vi "Translate.vi"(0 "Speed":i16, 11 "Turn":i16) -> (4 "Right Motor Speed":i16, 15 "Left Motor Speed":i16)   [LabVIEW 2009]
doc: "This VI takes in Speed and Turn values and converts them into wheel speeds.\nNOTE : Turn value of 0 indicates that the robot will go straight"
panel:
  in  "Min axix turn speed":i16=6
  in  "Max axix turn speed":i16=30
  in  "Wheel Diameter 2":dbl=0.4191 caption="Wheel Diameter=r(m)"
  out "Global wl":dbl
  out "Global wr":dbl
  out "wl":dbl caption="Left wheel angular velocity=wl(R/s)"
  out "wr":dbl caption="Right wheel angular velocity=wr(R/s)"
  in  "Wheel Diameter":dbl=0.21 caption="Wheel Radius=r(m)"
  in  "Distance Between wheels":dbl=0.6096 caption="Distance between wheels=L(m)"
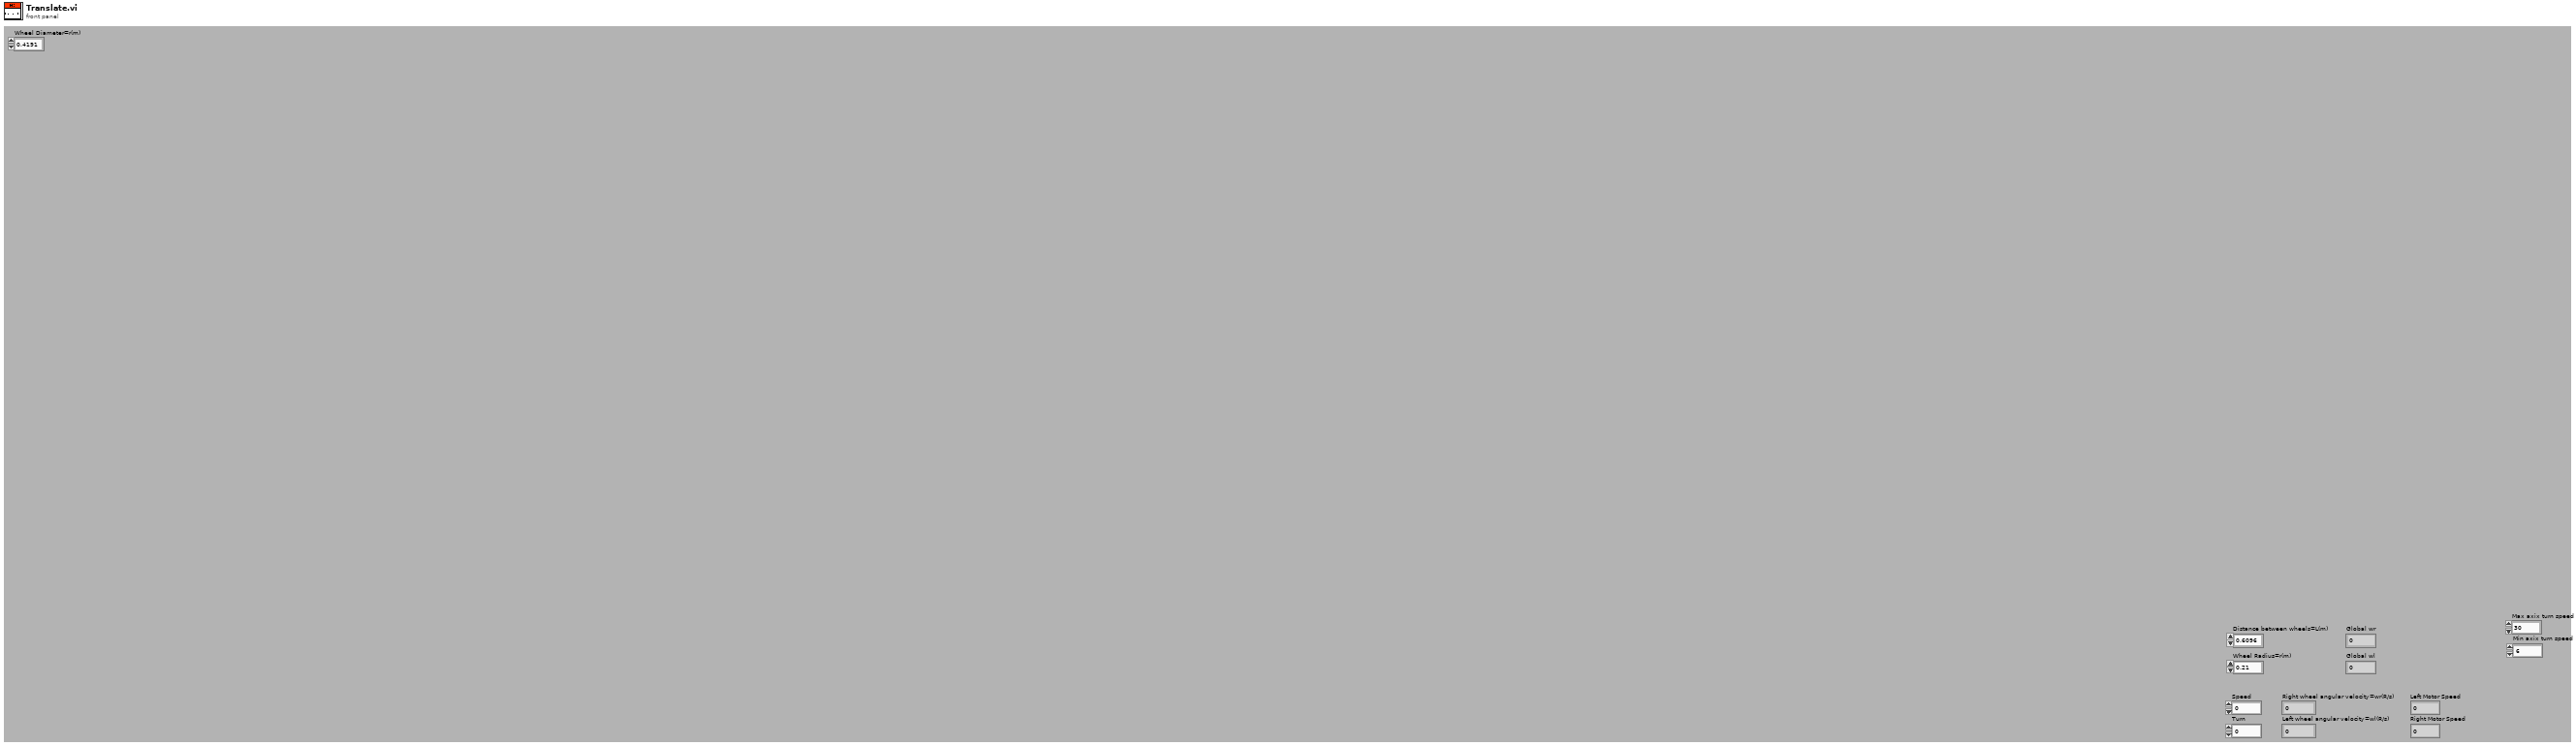
[diagram p1: front panel]
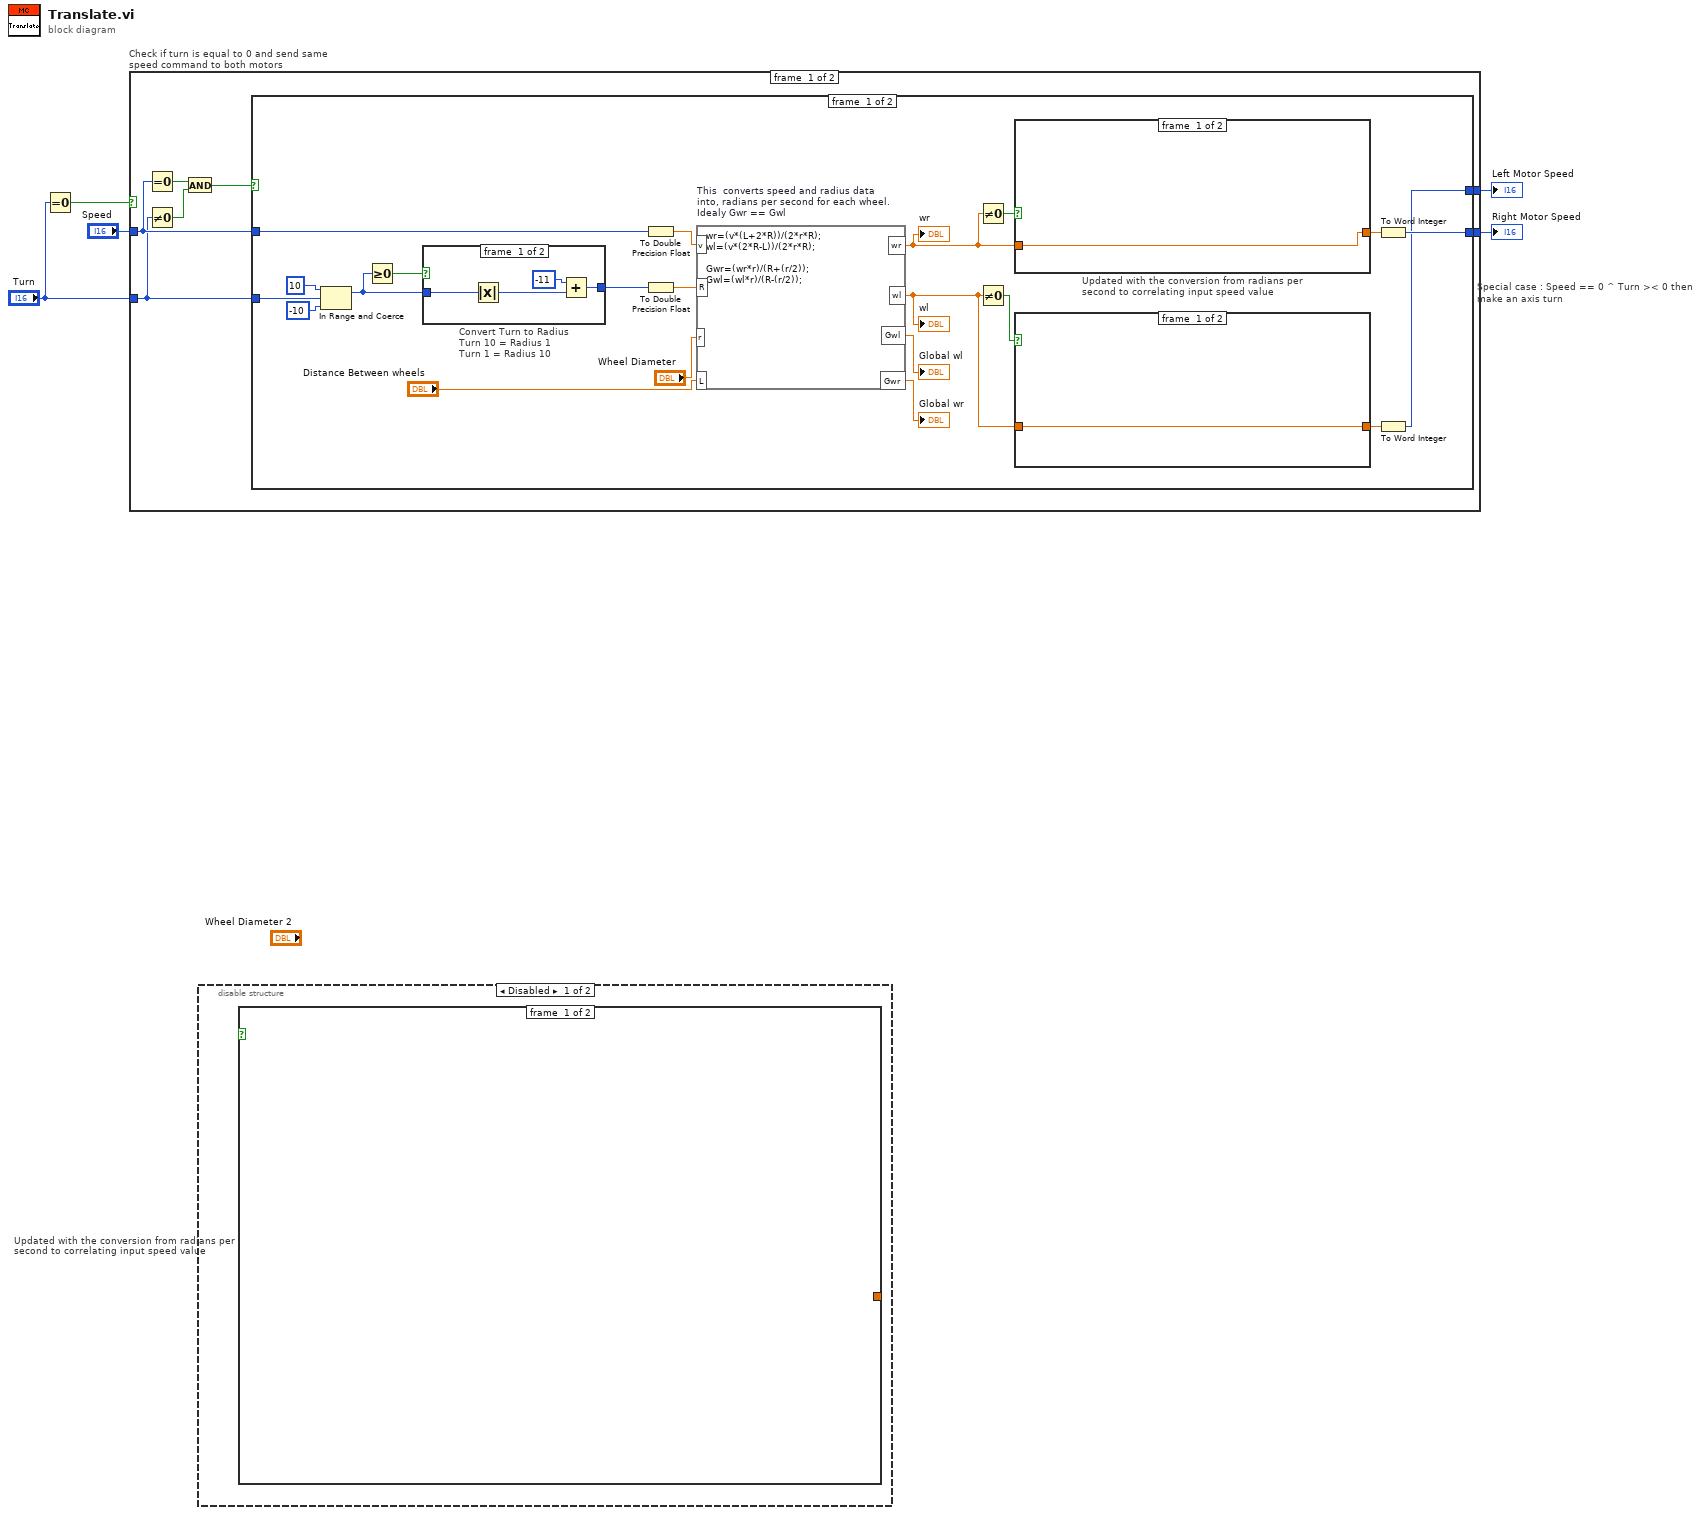
[diagram p0: block diagram]
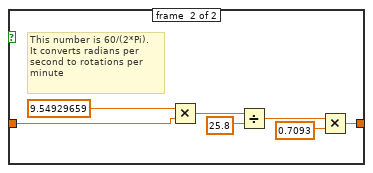
[diagram p2: hidden frame]
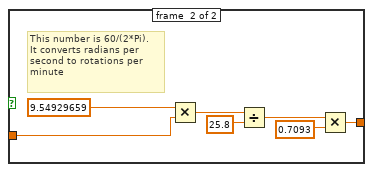
[diagram p3: hidden frame]
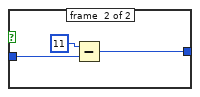
[diagram p4: hidden frame]
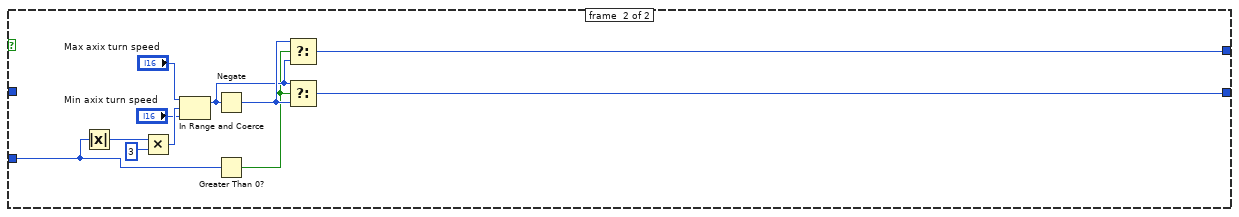
[diagram p5: hidden frame]
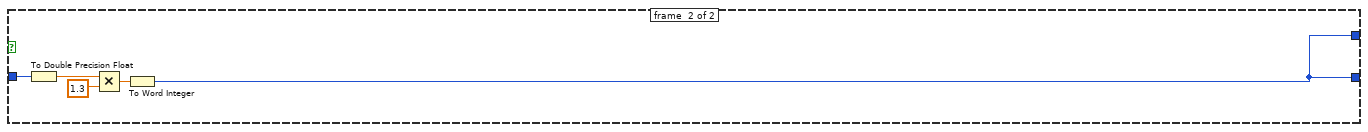
[diagram p6: hidden frame]
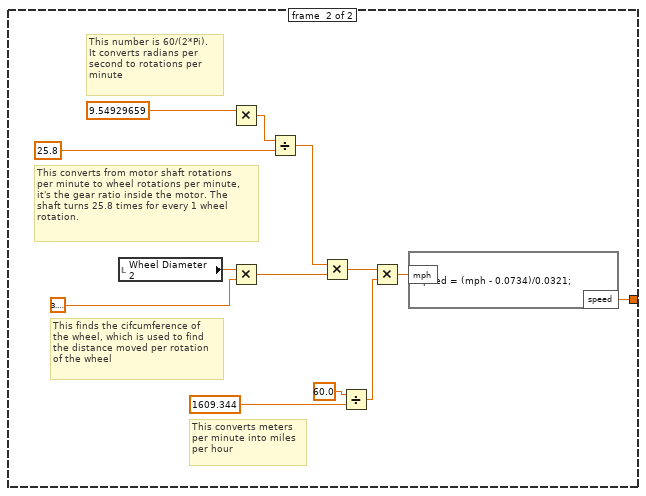
[diagram p7: hidden frame]
diagram:
  n1 = Equal To 0?(x="Turn") -> (x = 0?=w4:bool)
  n2 = case "Check if turn is equal to 0 and send same speed command to both motors" shown="False" w4 {
    tunnel: "Turn" -> [w8 _]
    tunnel: "Speed" -> [w10 w72]
    tunnel: [w12 w69] -> w2
    tunnel: [w11 w69] -> w1
    frame #0 {
      n3 = Equal To 0?(x=w10) -> (x = 0?=w9:bool)
      n4 = Not Equal To 0?(x=w8) -> (x != 0?=w6:bool)
      n5 = And(x=w9, y=w6) -> (x .and. y?=w7:bool)
      n6 = case "Special case : Speed == 0 ^ Turn >< 0 then make an axis turn" shown="False" w7 {
        tunnel: w8 -> [w27 w65]
        tunnel: w10 -> [w17 _]
        tunnel: [w15 w67] -> w12
        tunnel: [w13 w66] -> w11
        frame #0 {
          n7 = In Range and Coerce(upper limit=i16 10, x=w27, lower limit=i16 -10) -> (coerced(x)=w24:i16)  [unwired: 1 out]
          n8 = Greater Or Equal To 0?(x=w24) -> (x >= 0?=w28:bool)
          n9 = case "Convert Turn to Radius\nTurn 10 = Radius 1\nTurn 1 = Radius 10" shown="False" w28 {
            tunnel: w24 -> [w51 w56]
            tunnel: [w50 w54] -> w23
            frame #0 {
              n10 = Absolute Value(x=w51) -> (abs(x)=w52:i16)
              n11 = Add(x=i16 -11, y=w52) -> (x+y=w50:i16)
            }
            frame #1 {
              n12 = Subtract(x=i16 11, y=w56) -> (x-y=w54:i16)
            }
          }
          n13 = To Double Precision Float(number=w17) -> (double precision float=w18:dbl)
          n14 = To Double Precision Float(number=w23) -> (double precision float=w29:dbl)
          n15 = formula code="wr=(v*(L+2*R))/(2*r*R);\nwl=(v*(2*R-L))/(2*r*R);\n\nGwr=(wr*r)/(R+(r/2));\nGwl=(wl*r)/(R-(r/2));" "This  converts speed and radius data \ninto, radians per second for each wheel.\nIdealy Gwr == Gwl"("v"=w18, "R"=w29, "r"="Wheel Diameter", "L"="Distance Between wheels") -> ("wr"=w21:dbl, "wl"=w19:dbl, "Gwr"=→"Global wr":dbl, "Gwl"=→"Global wl":dbl)
          "wr" <- w21
          "wl" <- w19
          n16 = Not Equal To 0?(x=w21) -> (x != 0?=w22:bool)
          n17 = Not Equal To 0?(x=w19) -> (x != 0?=w20:bool)
          n18 = case "Updated with the conversion from radians per second to correlating input speed value" shown="True" w22 {
            tunnel: w21 -> [w42 w44]
            tunnel: [w42 w43] -> w16
            frame #0 {
            }
            frame #1 {
              # "This number is 60/(2*Pi). \nIt converts radians per \nsecond to rotations per \nminute"
              n19 = Multiply(x=9.54929659, y=w44) -> (x*y=w47:dbl)
              n20 = Divide(x=w47, y=25.8) -> (x/y=w45:dbl)
              n21 = Multiply(x=w45, y=0.7093 ("x")) -> (x*y=w43:dbl)
            }
          }
          n22 = case shown="True" w20 {
            tunnel: w19 -> [w34 w36]
            tunnel: [w34 w35] -> w14
            frame #0 {
            }
            frame #1 {
              # "This number is 60/(2*Pi). \nIt converts radians per \nsecond to rotations per \nminute"
              n23 = Multiply(x=9.54929659, y=w36) -> (x*y=w39:dbl)
              n24 = Divide(x=w39, y=25.8) -> (x/y=w37:dbl)
              n25 = Multiply(x=w37, y=0.7093 ("x")) -> (x*y=w35:dbl)
            }
          }
          n26 = To Word Integer(number=w16) -> (16bit integer=w15:i16)
          n27 = To Word Integer(number=w14) -> (16bit integer=w13:i16)
        }
        frame #1 {
          n28 = Absolute Value(x=w65) -> (abs(x)=w63:i16)
          n29 = Multiply(x=w63, y=i16 3) -> (x*y=w61:i16)
          n30 = In Range and Coerce(upper limit="Max axix turn speed", x=w61, lower limit="Min axix turn speed") -> (coerced(x)=w60:i16)  [unwired: 1 out]
          n31 = Negate(x=w60) -> (-x=w62:i16)
          n32 = Greater Than 0?(x=w65) -> (x > 0?=w57:bool)
          n33 = Select(t=w62, s=w57, f=w60) -> (s? t:f=w66:i16)
          n34 = Select(t=w60, s=w57, f=w62) -> (s? t:f=w67:i16)
        }
      }
    }
    frame #1 {
      n35 = To Double Precision Float(number=w72) -> (double precision float=w68:dbl)
      n36 = Multiply(x=w68, y=1.3) -> (x*y=w70:dbl)
      n37 = To Word Integer(number=w70) -> (16bit integer=w69:i16)
    }
  }
  "Right Motor Speed" <- w2
  "Left Motor Speed" <- w1
  n38 = disable-structure shown="Disabled" {
    frame #0 {
      n39 = case "Updated with the conversion from radians per second to correlating input speed value" shown="True" {
        selector: _ -> [_ _]
        tunnel: [_ w73] -> _
        frame #0 {
        }
        frame #1 {
          # "This converts meters\nper minute into miles\nper hour"
          # "This finds the cifcumference of\nthe wheel, which is used to find \nthe distance moved per rotation\nof the wheel"
          # "This converts from motor shaft rotations \nper minute to wheel rotations per minute,\nit's the gear ratio inside the motor. The \nshaft turns 25.8 times for every 1 wheel \nrotation."
          # "This number is 60/(2*Pi). \nIt converts radians per \nsecond to rotations per \nminute"
          n40 = local read "Wheel Diameter 2"() -> (w80:dbl)
          n41 = Multiply(x=9.54929659) -> (x*y=w84:dbl)  [unwired: 1 in]
          n42 = Multiply(x=w80, y=3.141592653589793) -> (x*y=w79:dbl)
          n43 = Divide(x=w84, y=25.8) -> (x/y=w82:dbl)
          n44 = Multiply(x=w82, y=w79) -> (x*y=w78:dbl)
          n45 = Divide(x=60.0, y=1609.344) -> (x/y=w75:dbl)
          n46 = Multiply(x=w78, y=w75) -> (x*y=w74:dbl)
          n47 = formula code="speed = (mph - 0.0734)/0.0321;"("mph"=w74) -> ("speed"=w73:dbl)
        }
      }
    }
    frame #1 {
    }
  }
